vi "Destroy.vi"(8 "Error In":errorcluster, 11 "reference in":refnum<class "MultiplicationHandler.lvclass">) -> (0 "Error Out":errorcluster, 3 "reference out":refnum<class "MultiplicationHandler.lvclass">)   [LabVIEW 2020, in "MultiplicationHandler.lvclass"]
uses:
  MultiplicationHandler.lvclass
  BaseHandler_class/BaseHandler.lvclass
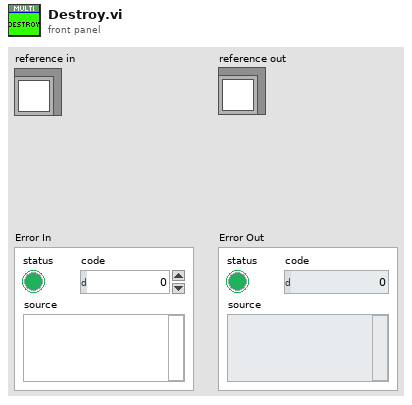
[diagram p1: front panel]
types:
  T1 = typedef "MultiplicationHandler.lvclass/ObjectAttributes.ctl" = cluster{"None":bool}
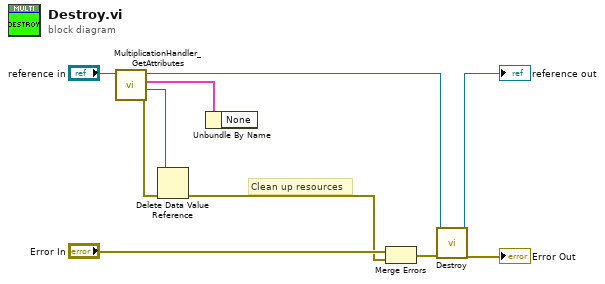
[diagram p0: block diagram]
diagram:
  # "Clean up resources"
  n1 = call "MultiplicationHandler_GetAttributes.vi"("reference in"="reference in") -> ("error out"=w8:errorcluster, "DataRef"=w5:refnum<data-value>, "Data"=w7:T1, "reference out"=w6:refnum<class "MultiplicationHandler.lvclass">)  [unwired: 7 in]
  n2 = Delete Data Value Reference(data value reference=w5, error in=w8) -> (error out=w3:errorcluster)  [unwired: 1 out]
  n3 = Unbundle By Name(w7) -> ()  [unwired: 1 out]
  n4 = Merge Errors("Error In", w3) -> (w10:errorcluster)
  n5 = call-parent "Destroy.vi"("Error In"=w10, "reference in"=w6) -> ("Error Out"=→"Error Out":errorcluster, "reference out"=→"reference out":refnum<class "MultiplicationHandler.lvclass">)  [unwired: 8 in]
